vi "Greatest Common Divisor (GCD)-scalar input.vi"(8 "error in (no error)":errorcluster, 10 "y":i32, 11 "x":i32) -> (0 "error out":errorcluster, 3 "Greatest Common Divisor (GCD)":i32)   [LabVIEW 2021, in "Numeric Utilities.lvlib"]
uses:
  Numeric Utilities.lvlib
panel:
  # "Development\ncontrols/indicators useful for development and testing, but which are not outputs of the VI"
  # "Input\nInputs to the VI"
  # "Output\nOutputs of the VI"
  # "Description\n\nBlank VI with error handling case. \n\nSummarize the use of this VI in this space."
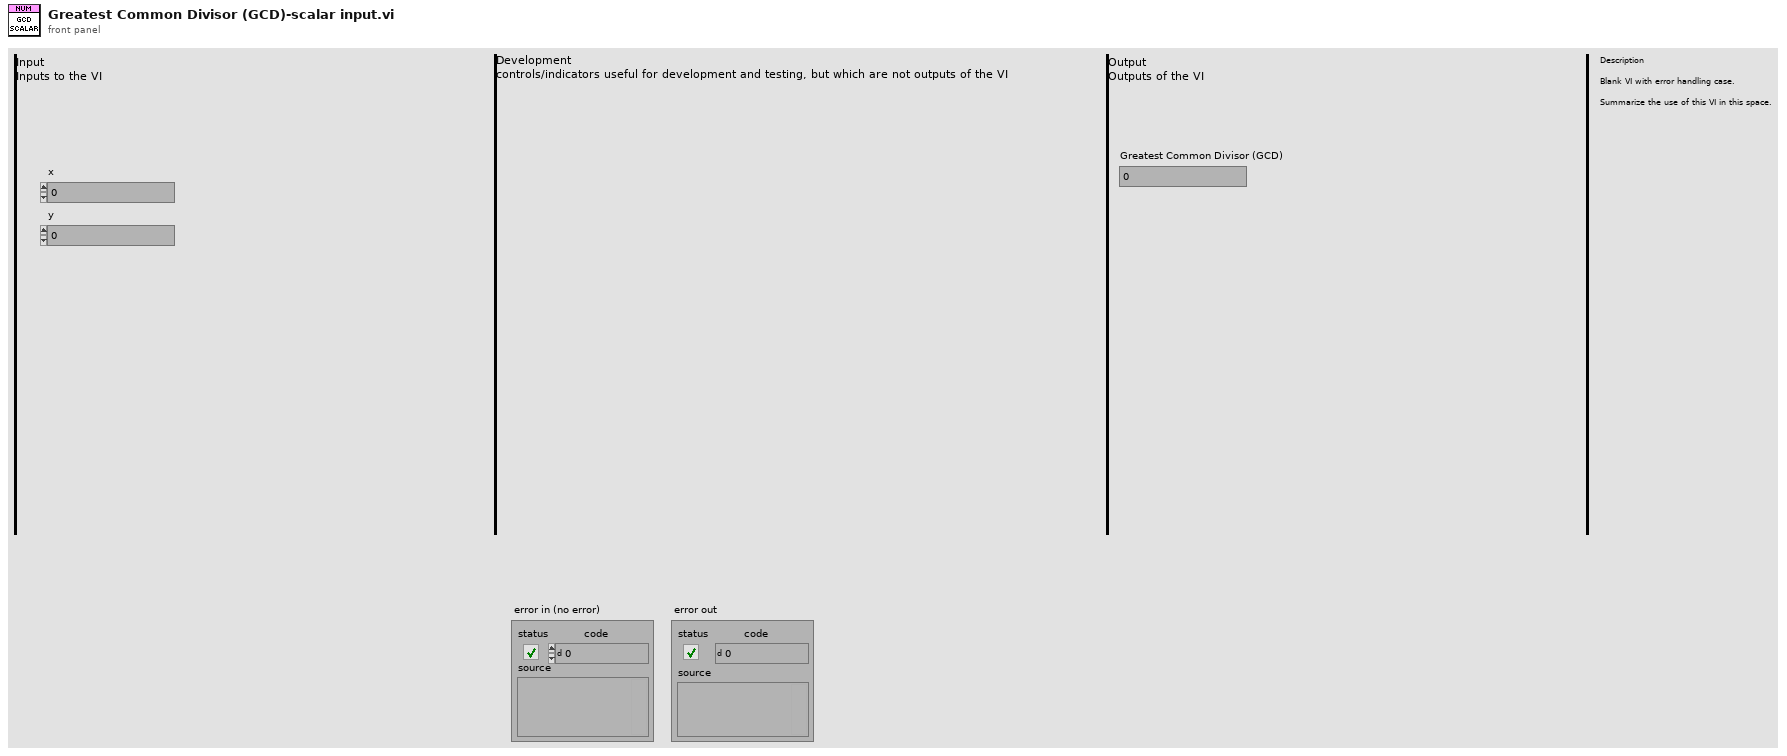
[diagram p1: front panel]
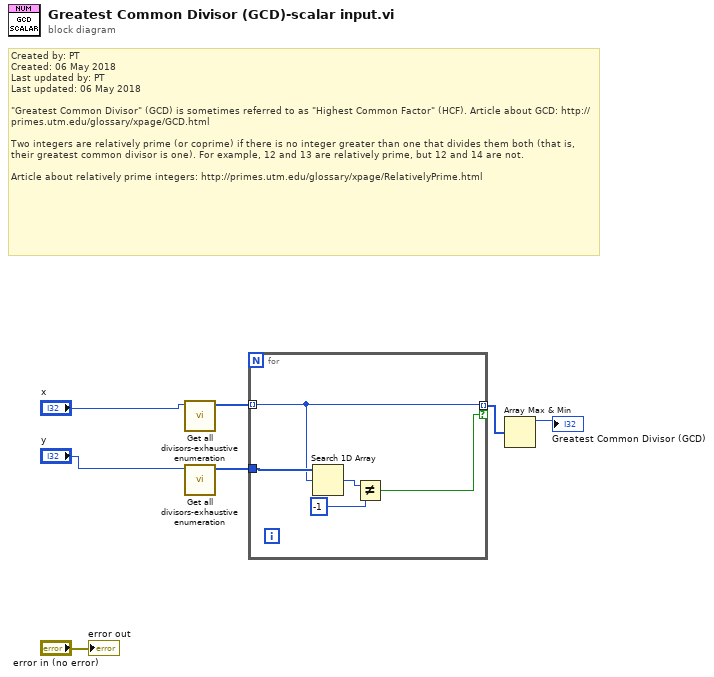
[diagram p0: block diagram]
diagram:
  # "Created by: PT\nCreated: 06 May 2018\nLast updated by: PT\nLast updated: 06 May 2018\n\n\"Greatest Common Divisor\" (GCD) is sometimes referred to as \"Highest Common Factor\" (HCF). Article about GCD: http://primes.utm.edu/glossary/xpage/GCD.html\n\nTwo integers are relatively prime (or coprime) if there is no integer greater than one that divides them both (that is, their greatest common divisor is one). For example, 12 and 13 are relatively prime, but 12 and 14 are not.\n\nArticle about relatively prime integers: http://primes.utm.edu/glossary/xpage/RelativelyPrime.html"
  n1 = call "Get all divisors-exhaustive enumeration.vi"("x"="x") -> ("Divisors"=w3:i32[])  [unwired: 7 in, 3 out]
  n2 = call "Get all divisors-exhaustive enumeration.vi"("x"="y") -> ("Divisors"=w2:i32[])  [unwired: 7 in, 3 out]
  n3 = for {
    tunnel: w3 -> [w9] mode=indexing
    tunnel: w2 -> [w12]
    tunnel: [w9] -> w1 mode=indexing if=w8
    n4 = Search 1D Array(1D array=w12, element=w9) -> (index of element=w11:i32)  [unwired: 1 in]
    n5 = Not Equal?(x=w11, y=-1) -> (x != y?=w8:bool)
  }
  n6 = Array Max & Min(array=w1) -> (max value=→"Greatest Common Divisor (GCD)":i32)  [unwired: 3 out]
  "error out" <- "error in (no error)"
